vi "MainForMerlin.vi"() -> ()   [LabVIEW 2018]
uses:
  classes/Tushars Events Toolkit/Software/Modules/EventClient_ObjectReference.ctl
  classes/Variable Manager/VariableManager_Bool.vi
  classes/Variable Manager/VariableManager_Double.vi
  <vilib>/Utility/file.llb/Write To Spreadsheet File (string).vi
  classes/Variable Manager/VariableManager_String.vi
  Strict Type Controls/Command.ctl
panel:
  out "filterSetup?":bool
  out "Quit":bool
  out "error out":errorcluster
  in  "error in (no error)":errorcluster
  in  "abort":bool
  in  "start":bool
  out "gratSetup?":bool
  out "statusFilter":bool
  in  "Start Filter":bool
  out "Agilent Current":dbl format="%#.4f A"
  out "Agilent Voltage":dbl format="%#.4f V"
  out "Test Status":bool
  out "statusMerlin":bool
  out "statusMC":bool
  out "statusPS":bool
  out "statusSM":bool
  in  "Start Merlin":bool
  in  "Start Monochromator":bool
  in  "Start Power Supply":bool
  in  "Start Source Meter":bool
  out "Merlin Voltage":dbl format="%#.7f mV"
  out "Measuring Wavelength":dbl format="%#.7f nm"
  out "Source Meter Voltage":dbl format="%#.7f mV"
  in  "Frequency":u32=8 min=8 max=1100 step=1
  in  "setMerlin":bool
  in  "#Filter":enum16{"None", "1 Pole", "2 Pole"}(ring)
  in  "Phase":enum16{"1 Phase", "2 Phase"}(ring)
  in  "SyncMode":T1(ring)
  in  "Time Const":T2(ring)
  in  "tab":T3(tab)=enum."Script"
  in  "exportVT":bool
  out "VTGraph":cluster{dbl[], dbl[]}(graph)
  in  "Test Mode":enum16{"Time Mode", "dV/dt Mode"}(ring)
  in  "Log Interval":u32=50 min=100 step=1 format="%.0f mSec"
  in  "Test Time":dbl step=1.0 format="%<%H:%M:%S>t"
  out "Time Remaining":dbl format="%<%H:%M:%S>t"
  in  "Target dV/dt":dbl format="%#.9f mV"
  in  "Lock In time":dbl step=1.0 format="%<%H:%M:%S>t"
  out "dV/dt":dbl format="%#.11f mV"
  out "Locked Time":dbl step=1.0 format="%<%H:%M:%S>t"
  in  "Perform Test After":T3(ring)=enum."Voltage Vs Wavelength"
  in  "setOffsets":bool
  in  "portD":bool
  in  "portA":bool
  in  "Settling Time (ms)":dbl=5000.0
  in  "To":dbl=1000.0
  in  "Step":dbl=100.0
  in  "From":dbl=100.0
  in  "exportSweep":bool
  out "sweep":cluster{dbl[], dbl[]}[](graph)
  in  "SetSlit":bool
  in  "SetGrating":bool
  in  "setWavelength":bool
  in  "Wavelength":dbl
  in  "Slit":string(combo)
  in  "GratingNo":u8=1 min=1 max=3 step=1
  in  "Sweep Results":i32(listbox)
  in  "exportScriptWave":bool
  out "scriptSweep":cluster{dbl[], dbl[]}[](graph)
  in  "Command":T4
  in  "Parm 4":dbl format="%#.6f"
  in  "Parm 3":dbl format="%#.6f"
  in  "openScript":bool
  in  "exportScript":bool
  in  "update":bool
  out "scriptGraph":cluster{dbl[], dbl[]}(graph)
  in  "Parm 2":dbl format="%#.6f"
  in  "Parm 1":dbl format="%#.6f"
  in  "script":i32(listbox)
  in  "add":bool
  in  "remove":bool
  in  "exportScriptResults":bool
  in  "Script Avg Interval":u32=200 min=100 step=1 format="%.0f mSec"
  # "Status"
  # "Merlin"
  # "Test Type"
  # "Test Time"
  # "Voltage Results"
  # "Monochromator"
  # "Merlin"
  # "Sweep"
  # "NOTE:\n1. if this LED is OFF then GPIB is not connected...\n2. Close program before power off Instruments..."
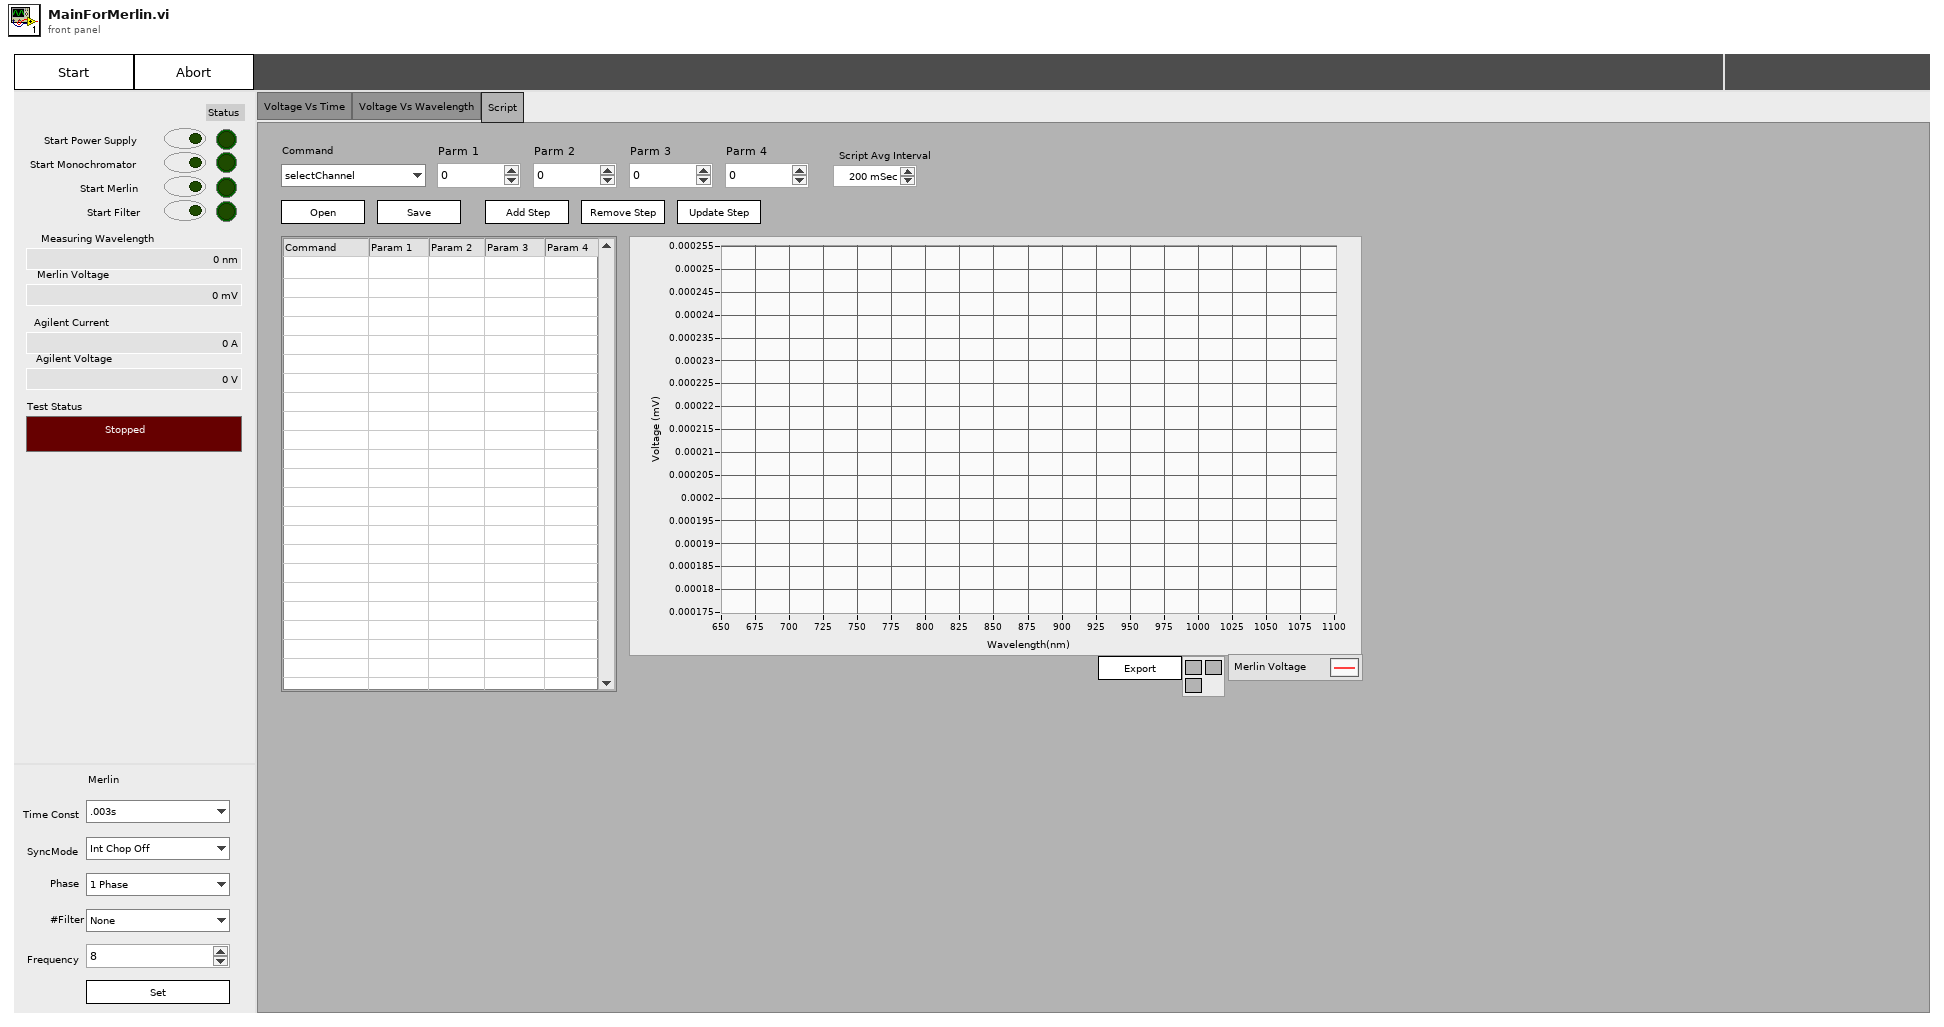
[diagram p1: front panel]
types:
  T1 = enum16{"Int Chop Off", "Int Chop On", "Ext Chop Off", "Ext Chop On"}
  T2 = enum16{".003s", ".010s", ".030s", ".100s", ".300s", "1.00s", "3.00s", "10.0s", "30.0s", "100s"}
  T3 = enum32{"Voltage Vs Time", "Voltage Vs Wavelength", "Script"}
  T4 = typedef "Command.ctl" = enum16{"selectChannel", "setDCVoltage", "setDCCurrent", "setVoltageSteps", "wait", "setWavelength", "setWavelengthSteps"}
  T5 = enum32{"invalid app kind", "Development System", "Run Time System", "Student Edition", "Embedded LabVIEW", "Evaluation", "Custom"}
  T6 = cluster{"startTime":u32, "lastUpdate":u32, "lastVoltage":dbl, "run?":bool, "From":dbl, "time":dbl[], "MerlinVal":dbl[], "SMVolt":dbl[], "sweepType":enum16{"ASC", "DESC"}, "Wavlnth":dbl[], "Test Mode":enum16{"Time Mode", "dV/dt Mode"}, "tab":enum32{"Voltage Vs Time", "Voltage Vs Wavelength", "Script"}, "script":string[][], "dV/dt":dbl[], "graphUpdate":u32}
  T7 = typedef "EventClient_ObjectReference.ctl" = refnum<k1>
  T8 = cluster{"#Stages":enum16{"None", "1 Pole", "2 Pole"}, "Phase":enum16{"1 Phase", "2 Phase"}, "SyncMode":enum16{"Int Chop Off", "Int Chop On", "Ext Chop Off", "Ext Chop On"}, "Time Const":enum16{".003s", ".010s", ".030s", ".100s", ".300s", "1.00s", "3.00s", "10.0s", "30.0s", "100s"}, "Frequency":u32}
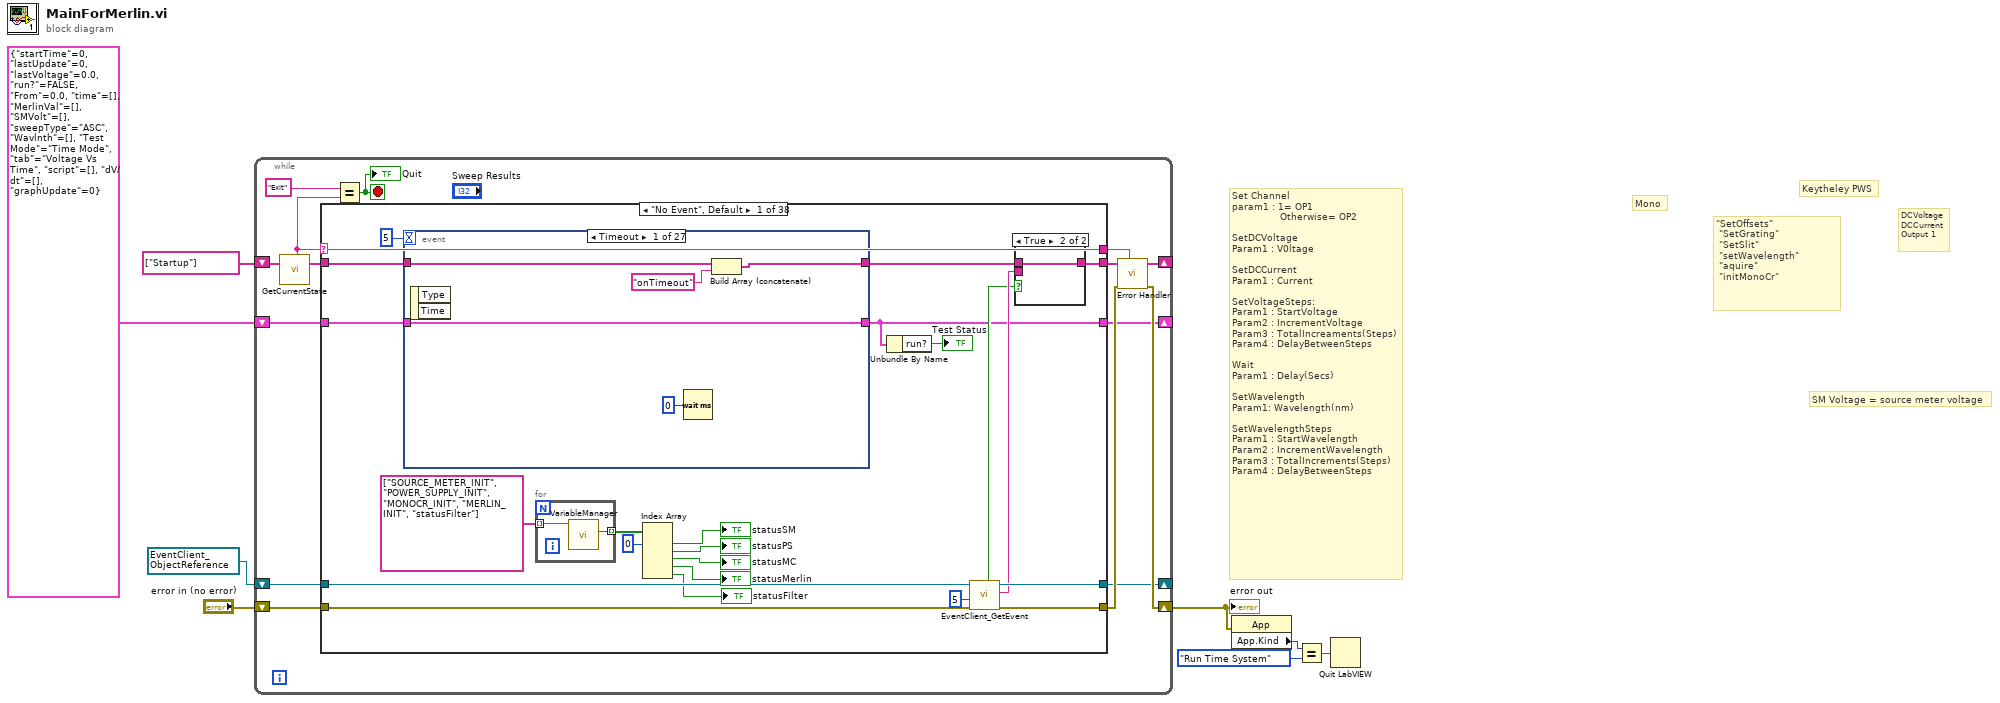
[diagram p0: block diagram]
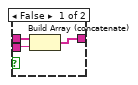
[diagram p2: hidden frame]
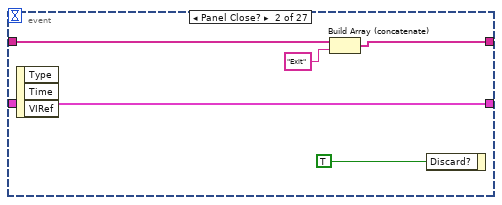
[diagram p3: hidden frame]
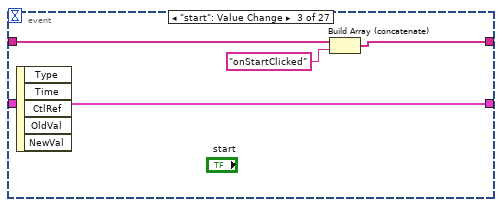
[diagram p4: hidden frame]
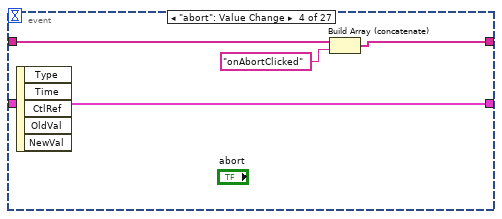
[diagram p5: hidden frame]
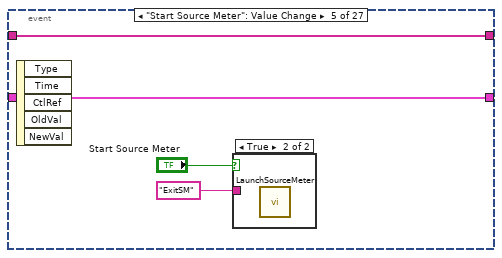
[diagram p6: hidden frame]
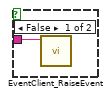
[diagram p7: hidden frame]
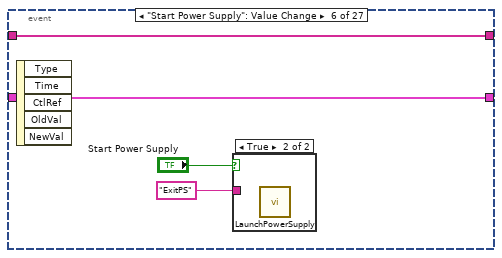
[diagram p8: hidden frame]
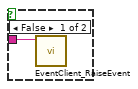
[diagram p9: hidden frame]
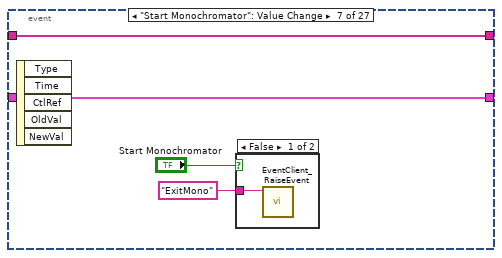
[diagram p10: hidden frame]
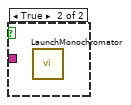
[diagram p11: hidden frame]
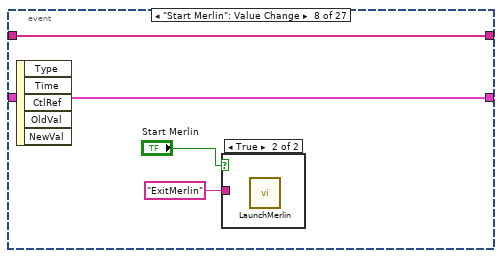
[diagram p12: hidden frame]
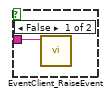
[diagram p13: hidden frame]
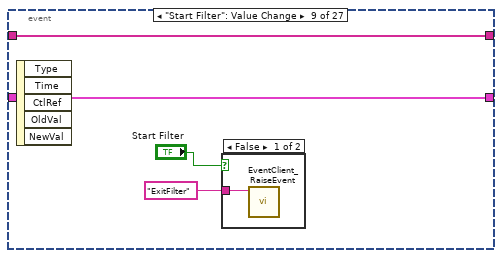
[diagram p14: hidden frame]
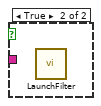
[diagram p15: hidden frame]
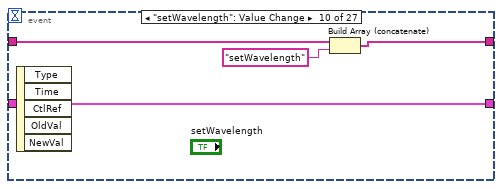
[diagram p16: hidden frame]
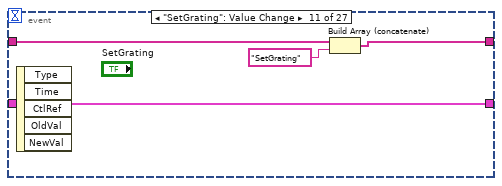
[diagram p17: hidden frame]
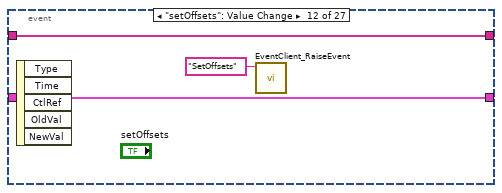
[diagram p18: hidden frame]
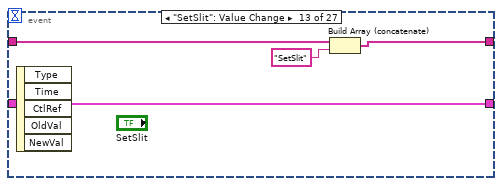
[diagram p19: hidden frame]
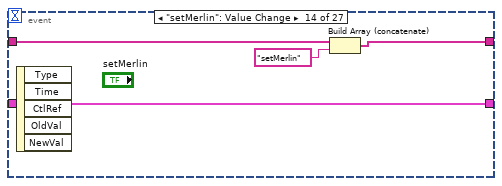
[diagram p20: hidden frame]
diagram:
  w7 = T7 refnum items=["EventClient"] ("reference")
  # "SM Voltage = source meter voltage"
  # "Keytheley PWS"
  # "Mono"
  # "DCVoltage\nDCCurrent\nOutput 1"
  # "\"SetOffsets\"\n \"SetGrating\"  \n \"SetSlit\"\n \"setWavelength\"\n \"aquire\"  \n \"initMonoCr\""
  # "Set Channel\nparam1 : 1= OP1\n                Otherwise= OP2\n\nSetDCVoltage\nParam1 : V0ltage\n\nSetDCCurrent\nParam1 : Current\n\nSetVoltageSteps:\nParam1 : StartVoltage\nParam2 : IncrementVoltage\nParam3 : TotalIncreaments(Steps)\nParam4 : DelayBetweenSteps\n\nWait\nParam1 : Delay(Secs)\n\nSetWavelength\nParam1: Wavelength(nm)\n\nSetWavelengthSteps\nParam1 : StartWavelength\nParam2 : IncrementWavelength\nParam3 : TotalIncrements(Steps)\nParam4 : DelayBetweenSteps"
  n1 = while {
    shift-right: [w19] -> _
    shift-left: string[] ["Startup"] ("State Array Out") -> [w23]
    shift-right: [w15] -> w4
    shift-left: "error in (no error)" -> [w16]
    shift-right: [w12] -> _
    shift-left: w7 -> [w11]
    shift-right: [w9] -> _
    shift-left: T6 {"startTime"=0, "lastUpdate"=0, "lastVoltage"=0.0, "run?"=FALSE, "From"=0.0, "time"=[], "MerlinVal"=[], "SMVolt"=[], "sweepType"=enum."ASC", "Wavlnth"=[], "Test Mode"=enum."Time Mode", "tab"=enum."Voltage Vs Time", "script"=[], "dV/dt"=[], "graphUpdate"=0} -> [w10]
    stop <- w20 stop-if-true
    n2 = call "GetCurrentState.vi"("State Array In"=w23) -> ("Current State"=w13:string, "State Array Out"=w22:string[])  [unwired: 17 in]
    n3 = case shown="\"No Event\", Default" w13 {
      selector: w13 -> [w46 w193 w202 w212 w230 w246 w269 w296 w315 w325 w346 w363 w371 w398 w414 w425 w437 w445 w449 w458 w467 w479 w487 w497 w526 w537 w542 w560 w612 w632 w662 w694 w719 w782 w837 w872 w901 w907]
      tunnel: w22 -> [w45 w192 w208 w213 w231 w247 w270 w297 w302 w326 w347 w364 w372 w399 w415 w426 w438 w446 w453 w462 w469 w483 w488 w498 w527 w538 w543 w551 w595 w616 w654 w686 w710 w783 w838 w873 w900 w904]
      tunnel: [w36 w191 w208 w213 w231 w247 w270 w297 w302 w326 w347 w364 w372 w399 w415 w426 w438 w446 w453 w462 w469 w483 w488 w498 w527 w538 w543 w552 w594 w615 w653 w688 w709 w783 w826 w873 w900 w904] -> w18
      tunnel: [w41 w185 w203 w211 w229 w245 w268 w295 w314 w324 w345 w362 w370 w397 w413 w424 w431 w439 w450 w459 w465 w480 w486 w493 w522 w533 w541 w559 w611 w631 w661 w693 w717 w764 w833 w871 w899 w906] -> w14
      tunnel: [w46 w193 w202 w212 w230 w246 w269 w296 w315 w325 w346 w363 w371 w398 w414 w425 w437 w445 w449 w458 w467 w479 w487 w497 w526 w537 w542 w560 w612 w632 w662 w694 w719 w782 w837 w872 w901 w907] -> w17
      tunnel: w16 -> [w42 w172 w206 w211 w229 w245 w268 w295 w314 w324 w345 w362 w370 w397 w413 w424 w432 w440 w451 w460 w464 w481 w486 w495 w524 w535 w541 w559 w611 w631 w661 w693 w717 w763 w834 w871 w899 w905]
      tunnel: [w40 w183 w205 w210 w228 w244 w267 w294 w313 w323 w344 w361 w369 w396 w412 w423 w436 w444 w452 w461 w468 w482 w485 w491 w520 w531 w540 w558 w610 w630 w660 w692 w718 w781 w836 w870 w898 w902] -> w12
      tunnel: w11 -> [w43 _ w207 w210 w228 w244 w267 w294 w313 w323 w344 w361 w369 w396 w412 w423 w436 w444 w452 w461 w468 w482 w485 w496 w525 w536 w540 w558 w610 w630 w660 w692 w718 w781 w836 w870 w898 w902]
      tunnel: w10 -> [w27 w181 w201 w209 w227 w243 w266 w293 w312 w322 w343 w360 w368 w395 w411 w422 w435 w443 w447 w457 w466 w472 w484 w489 w519 w530 w539 w557 w600 w629 w658 w691 w712 w780 w824 w863 w897 w903]
      tunnel: [w26 w181 w201 w209 w227 w243 w266 w293 w312 w322 w343 w360 w368 w394 w410 w422 w435 w443 w447 w457 w466 w472 w484 w489 w519 w530 w539 w557 w599 w626 w656 w691 w711 w779 w835 w862 w897 w903] -> w9
      frame "No Event", Default {
        n4 = event shown="[0] Timeout" {
          selector: _ -> [_ _ _ _ _ _ _ _ _ _ _ _ _ _ _ _ _ _ _ _ _ _ _ _ _ _ _]
          dyn-events: _ -> [_ _ _ _ _ _ _ _ _ _ _ _ _ _ _ _ _ _ _ _ _ _ _ _ _ _ _]
          timeout: 5 -> [_ _ _ _ _ _ _ _ _ _ _ _ _ _ _ _ _ _ _ _ _ _ _ _ _ _ _]
          tunnel: [w55 w60 w65 w69 w74 w79 w84 w89 w94 w98 w102 w105 w109 w113 w117 w121 w125 w129 w133 w137 w141 w145 w149 w153 w157 w161 w166] -> w37
          tunnel: w45 -> [w57 w62 w66 w70 w74 w79 w84 w89 w94 w99 w103 w105 w110 w114 w118 w122 w126 w130 w134 w138 w142 w146 w150 w154 w158 w162 w166]
          tunnel: w27 -> [w56 w58 w63 w67 w73 w78 w83 w88 w93 w96 w100 w106 w107 w111 w115 w119 w123 w127 w131 w135 w139 w143 w147 w151 w155 w159 w167]
          tunnel: [w56 w58 w63 w67 w73 w78 w83 w88 w93 w96 w100 w106 w107 w111 w115 w119 w123 w127 w131 w135 w139 w143 w147 w151 w155 w159 w167] -> w26
          event Timeout {
            n5 = event-data() -> ()  [unwired: 1 in, 2 out]
            n6 = Wait (ms)(milliseconds to wait=u32 0) -> ()  [unwired: 1 out]
            n7 = Build Array (concatenate)(w57, "onTimeout" ("x")) -> (w55:string[])
          }
          event Panel Close? {
            n8 = event-data() -> ()  [unwired: 1 in, 3 out]
            n9 = Build Array (concatenate)(w62, "Exit" ("x")) -> (w60:string[])
            n10 = event-data("Discard?"=TRUE) -> ()  [unwired: 1 in, 1 out]
          }
          event "start": Value Change {
            n11 = event-data() -> ()  [unwired: 1 in, 5 out]
            n12 = Build Array (concatenate)(w66, "onStartClicked" ("x")) -> (w65:string[])
          }
          event "abort": Value Change {
            n13 = event-data() -> ()  [unwired: 1 in, 5 out]
            n14 = Build Array (concatenate)(w70, "onAbortClicked" ("x")) -> (w69:string[])
          }
          event "Start Source Meter": Value Change {
            n15 = event-data() -> ()  [unwired: 1 in, 5 out]
            n16 = case shown="True" "Start Source Meter" {
              tunnel: "ExitSM" -> [w75 _]
              frame False {
                n17 = call "EventClient_RaiseEvent.vi"("Event"=w75) -> ()  [unwired: 10 in, 1 out]
              }
              frame True {
                n18 = call "LaunchSourceMeter.vi"() -> ()  [unwired: 11 in, 1 out]
              }
            }
          }
          event "Start Power Supply": Value Change {
            n19 = event-data() -> ()  [unwired: 1 in, 5 out]
            n20 = case shown="True" "Start Power Supply" {
              tunnel: "ExitPS" -> [w80 _]
              frame False {
                n21 = call "EventClient_RaiseEvent.vi"("Event"=w80) -> ()  [unwired: 10 in, 1 out]
              }
              frame True {
                n22 = call "LaunchPowerSupply.vi"() -> ()  [unwired: 11 in, 1 out]
              }
            }
          }
          event "Start Monochromator": Value Change {
            n23 = event-data() -> ()  [unwired: 1 in, 5 out]
            n24 = case shown="False" "Start Monochromator" {
              tunnel: "ExitMono" -> [w85 _]
              frame False {
                n25 = call "EventClient_RaiseEvent.vi"("Event"=w85) -> ()  [unwired: 10 in, 1 out]
              }
              frame True {
                n26 = call "LaunchMonochromator.vi"() -> ()  [unwired: 11 in, 1 out]
              }
            }
          }
          event "Start Merlin": Value Change {
            n27 = event-data() -> ()  [unwired: 1 in, 5 out]
            n28 = case shown="True" "Start Merlin" {
              tunnel: "ExitMerlin" -> [w90 _]
              frame False {
                n29 = call "EventClient_RaiseEvent.vi"("Event"=w90) -> ()  [unwired: 10 in, 1 out]
              }
              frame True {
                n30 = call "LaunchMerlin.vi"() -> ()  [unwired: 11 in, 1 out]
              }
            }
          }
          event "Start Filter": Value Change {
            n31 = event-data() -> ()  [unwired: 1 in, 5 out]
            n32 = case shown="False" "Start Filter" {
              tunnel: "ExitFilter" -> [w95 _]
              frame False {
                n33 = call "EventClient_RaiseEvent.vi"("Event"=w95) -> ()  [unwired: 10 in, 1 out]
              }
              frame True {
                n34 = call "LaunchFilter.vi"() -> ()  [unwired: 11 in, 1 out]
              }
            }
          }
          event "setWavelength": Value Change {
            n35 = event-data() -> ()  [unwired: 1 in, 5 out]
            n36 = Build Array (concatenate)(w99, "setWavelength" ("x")) -> (w98:string[])
          }
          event "SetGrating": Value Change {
            n37 = event-data() -> ()  [unwired: 1 in, 5 out]
            n38 = Build Array (concatenate)(w103, "SetGrating" ("x")) -> (w102:string[])
          }
          event "setOffsets": Value Change {
            n39 = event-data() -> ()  [unwired: 1 in, 5 out]
            n40 = call "EventClient_RaiseEvent.vi"("Event"="SetOffsets") -> ()  [unwired: 10 in, 1 out]
          }
          event "SetSlit": Value Change {
            n41 = event-data() -> ()  [unwired: 1 in, 5 out]
            n42 = Build Array (concatenate)(w110, "SetSlit" ("x")) -> (w109:string[])
          }
          event "setMerlin": Value Change {
            n43 = event-data() -> ()  [unwired: 1 in, 5 out]
            n44 = Build Array (concatenate)(w114, "setMerlin" ("x")) -> (w113:string[])
          }
          event "exportSweep": Value Change {
            n45 = event-data() -> ()  [unwired: 1 in, 5 out]
            n46 = Build Array (concatenate)(w118, "exportSweep" ("x")) -> (w117:string[])
          }
          event "exportVT": Value Change {
            n47 = event-data() -> ()  [unwired: 1 in, 5 out]
            n48 = Build Array (concatenate)(w122, "exportVT" ("x")) -> (w121:string[])
          }
          event "portA": Value Change {
            n49 = event-data() -> ()  [unwired: 1 in, 5 out]
            n50 = Build Array (concatenate)(w126, "portA" ("x")) -> (w125:string[])
          }
          event "portD": Value Change {
            n51 = event-data() -> ()  [unwired: 1 in, 5 out]
            n52 = Build Array (concatenate)(w130, "portD" ("x")) -> (w129:string[])
          }
          event "add": Value Change {
            n53 = event-data() -> ()  [unwired: 1 in, 5 out]
            n54 = Build Array (concatenate)(w134, "addStep" ("x")) -> (w133:string[])
          }
          event "remove": Value Change {
            n55 = event-data() -> ()  [unwired: 1 in, 5 out]
            n56 = Build Array (concatenate)(w138, "removeStep" ("x")) -> (w137:string[])
          }
          event "update": Value Change {
            n57 = event-data() -> ()  [unwired: 1 in, 5 out]
            n58 = Build Array (concatenate)(w142, "updateStep" ("x")) -> (w141:string[])
          }
          event "exportScript": Value Change {
            n59 = event-data() -> ()  [unwired: 1 in, 5 out]
            n60 = Build Array (concatenate)(w146, "exportScript" ("x")) -> (w145:string[])
          }
          event "exportScriptResults": Value Change {
            n61 = event-data() -> ()  [unwired: 1 in, 5 out]
            n62 = Build Array (concatenate)(w150, "exportScriptResults" ("x")) -> (w149:string[])
          }
          event "exportScriptWave": Value Change {
            n63 = event-data() -> ()  [unwired: 1 in, 5 out]
            n64 = Build Array (concatenate)(w154, "exportScriptWave" ("x")) -> (w153:string[])
          }
          event "openScript": Value Change {
            n65 = event-data() -> ()  [unwired: 1 in, 5 out]
            n66 = Build Array (concatenate)(w158, "openScript" ("x")) -> (w157:string[])
          }
          event "script": Value Change {
            n67 = event-data() -> ()  [unwired: 1 in, 5 out]
            n68 = Build Array (concatenate)(w162, "onScriptRowSelected" ("x")) -> (w161:string[])
          }
          event Value Change {
            n69 = event-data() -> ("NewVal"=w164:T4)  [unwired: 1 in, 4 out]
            n70 = Index Array(array=string[] ["Set Channel\nparam1 : \n1                 = OP1\nOtherwise = OP2", "SetDCVoltage\nParam1 : V0ltage", "SetDCCurrent\nParam1 : Current", "SetVoltageSteps:\nParam1 : StartVoltage\nParam2 : IncrementVoltage\nParam3 : TotalIncreaments(Steps)\nParam4 : DelayBetweenSteps", "Wait\nParam1 : Delay(Secs)", "SetWavelength\nParam1: Wavelength(nm)", "SetWavelengthSteps\nParam1 : StartWavelength\nParam2 : IncrementWavelength\nParam3 : TotalIncrements(Steps)\nParam4 : DelayBetweenSteps"] ("Array"), index=w164) -> (element=w165:string)
            n71 = property on="Command" class="Enum (strict)"("TipStrip"=w165) -> ()  [unwired: 2 in, 2 out]
          }
        }
        n72 = for {
          tunnel: string[] ["SOURCE_METER_INIT", "POWER_SUPPLY_INIT", "MONOCR_INIT", "MERLIN_INIT", "statusFilter"] ("State Array Out") -> [w48] mode=indexing
          tunnel: [w47] -> w33 mode=indexing
          n73 = call-poly "VariableManager.vi"("Tag"=w48) -> ("Value out"=w47:bool)  [unwired: 7 in, 3 out]
        }
        n74 = Index Array(array=w33, index #1=0 ("index")) -> (element #1=→"statusSM":bool, element #2=→"statusPS":bool, element #3=→"statusMC":bool, element #4=→"statusMerlin":bool, element #5=→"statusFilter":bool)  [unwired: 4 in]
        n75 = Unbundle By Name(w26) -> ("run?"=→"Test Status":bool)
        n76 = call "EventClient_GetEvent.vi"("error in (no error)"=w42, "timeout in ms (-1)"=5, "reference"=w43) -> ("error out"=w41:errorcluster, "Name"=w39:string, "reference out"=w40:T7, "timed out?"=w38:bool)  [unwired: 4 in, 1 out]
        n77 = case shown="True" w38 {
          tunnel: w37 -> [w51 w52]
          tunnel: w39 -> [w50 _]
          tunnel: [w49 w52] -> w36
          frame False {
            n78 = Build Array (concatenate)(w51, w50) -> (w49:string[])
          }
          frame True {
          }
        }
      }
      frame "Startup" {
        w170 = cluster{dbl[], dbl[]}[] [] ("sweep")
        w171 = cluster{dbl[], dbl[]} {[], []} ("VTGraph")
        w175 = string[] ["Command", "Param 1", "Param 2", "Param 3", "Param 4"]  # script
        w176 = FALSE ("Start Source Meter")
        w169 = u32 200 ("Log Interval")
        # "If Multiple instnances of this VI are possible \nthen make sure that client created in each instance gets a different Name"
        n79 = local write "Log Interval"(w169) -> ()
        n80 = local write "Target dV/dt"(1.0 ("Target dV/dt")) -> ()
        n81 = local write "Lock In time"(30.0 ("Lock In time")) -> ()
        n82 = local write "sweep"(w170) -> ()
        n83 = local write "Test Time"(90.0 ("Locked Time")) -> ()
        n84 = local write "VTGraph"(w171) -> ()
        n85 = local write "scriptGraph"(w171) -> ()
        n86 = local write "Script Avg Interval"(w169) -> ()
        n87 = disable-structure shown="Disabled" {
          disable-tunnel: [w200 _] -> w177
          disable-tunnel: w172 -> [w199 _]
          frame Disabled {
            n88 = call "LaunchPowerSupply.vi"("error in (no error)"=w199) -> ("error out"=w198:errorcluster)  [unwired: 10 in]
            n89 = call "LaunchSourceMeter.vi"("error in (no error)"=w198) -> ("error out"=w197:errorcluster)  [unwired: 10 in]
            n90 = call "LaunchMerlin.vi"("error in (no error)"=w197) -> ("error out"=w196:errorcluster)  [unwired: 10 in]
            n91 = call "LaunchMonochromator.vi"("error in (no error)"=w196) -> ("error out"=w200:errorcluster)  [unwired: 10 in]
          }
          frame Enabled {
          }
        }
        n92 = local write "scriptSweep"(w170) -> ()
        n93 = local write "tab"(T3."Voltage Vs Wavelength" ("tab")) -> ()
        n94 = for {
          tunnel: bool[] [FALSE, TRUE] -> [w194] mode=indexing
          i -> [w195]
          n95 = property on="sweep" class="XYGraph (strict)"("Active Plot"=w195, "Plot.Visible?"=w194) -> ()  [unwired: 2 in, 2 out]
          n96 = property on="scriptSweep" class="XYGraph (strict)"("Active Plot"=w195, "Plot.Visible?"=w194) -> ()  [unwired: 2 in, 2 out]
        }
        n97 = Build Array (concatenate)(w192, string[] [] ("State Array Out")) -> (w191:string[])
        n98 = Call Chain() -> (call chain=w189:string[])
        n99 = Index Array(array=w189, index=0) -> (element=w187:string)
        n100 = call "EventClient_Create.vi"("error in (no error)"=w177, "Instance Name"=w187) -> ("error out"=w186:errorcluster, "reference"=w184:T7)  [unwired: 8 in]
        n101 = local write "Start Source Meter"(w176) -> ()
        n102 = local write "Start Power Supply"(w176) -> ()
        n103 = local write "Start Monochromator"(w176) -> ()
        n104 = local write "Start Merlin"(w176) -> ()
        n105 = call "EventClient_SubscribeEvents.vi"("error in (no error)"=w186, "Events"=string[] ["currGrating", "updateScriptSweep"], "reference"=w184) -> ("error out"=w185:errorcluster, "reference out"=w183:T7)  [unwired: 7 in]
        n106 = property on="script" class="MCListbox (strict)"("ColHdrString"=w175, "ItemNames"=string[][] [] ("Item Names")) -> ()  [unwired: 2 in, 2 out]
      }
      frame "Exit" {
        w205 = T7 refnum items=["EventClient"] ("reference out")
        n107 = call "EventClient_Destroy.vi"("error in (no error)"=w206, "reference"=w207) -> ("error out"=w204:errorcluster)  [unwired: 9 in]
        n108 = call "EventClient_RaiseEvent.vi"("error in (no error)"=w204, "Event"=w202) -> ("error out"=w203:errorcluster)  [unwired: 9 in]
      }
      frame "---------------Below are UI Events---------------" {
        # "This State will never Execute\nIt is added just for improving code readability please do not remove this case"
      }
      frame "onScriptRowSelected" {
        w219 = 0 ("index")
        n109 = property on="script" class="MCListbox (strict)"() -> ("ItemNames"=w226:string[][], "Value"=w225:i32)  [unwired: 2 in, 2 out]
        n110 = Index Array(array=w226, index (row)=w225) -> (element=w223:string[])  [unwired: 1 in]
        n111 = Delete From Array(array=w223, index=w219) -> (deleted portion=w222:string, array with subset deleted=w224:string[])  [unwired: 1 in]
        n112 = Scan From String(input string=w222, default 1=Command."selectChannel" ("Command")) -> (output 1=w218:T4)  [unwired: 3 in, 3 out]
        n113 = Fract/Exp String To Number(string=w224) -> (number=w220:dbl[])  [unwired: 3 in, 1 out]
        n114 = Index Array(array=w220, index #1=w219) -> (element #1=w217:dbl, element #2=w216:dbl, element #3=w215:dbl, element #4=w214:dbl)  [unwired: 3 in]
        n115 = local write "Parm 1"(w217) -> ()
        n116 = local write "Parm 2"(w216) -> ()
        n117 = local write "Parm 3"(w215) -> ()
        n118 = local write "Parm 4"(w214) -> ()
        n119 = local write "Command"(w218) -> ()
      }
      frame "exportVT" {
        n120 = local read "VTGraph"() -> (w237:cluster{dbl[], dbl[]})
        n121 = Unbundle(w237) -> (w241:dbl[], w238:dbl[])
        n122 = for {
          tunnel: w241 -> [w252] mode=indexing
          tunnel: "%<%H:%M:%S>t" ("format string") -> [w254]
          tunnel: [w253] -> w240 mode=indexing
          n123 = Format Into String(format string=w254, w252) -> (resulting string=w253:string)  [unwired: 2 in, 1 out]
        }
        n124 = Number To Fractional String(number=w238) -> (F-format string=w239:string[])  [unwired: 3 in]
        n125 = Build Array(w240, w239) -> (w236:string[][])
        n126 = Transpose 2D Array(2D array=w236) -> (transposed array=w232:string[][])
        n127 = call "File Dialog2"("pattern (all files)"="*.csv") -> ("selected path"=w235:path, "error out"=w234:errorcluster)  [unwired: 11 in, 2 out]
        n128 = case shown="Error" w234 {
          selector: w234 -> [_ w251]
          tunnel: w235 -> [w249 _]
          tunnel: w232 -> [w248 _]
          frame No Error {
            n129 = call-poly <vilib>:"Write To Spreadsheet File.vi"("delimiter (\\t)"="," ("delimiter (\\t)"), "2D data"=w248, "file path (dialog if empty)"=w249) -> ()  [unwired: 5 in, 1 out]
          }
          frame Error {
            n130 = call <vilib>:"Clear Errors.vi"("error in (no error)"=w251) -> ()  [unwired: 5 in, 2 out]
          }
        }
      }
      frame "exportScriptResults" {
        n131 = local read "scriptGraph"() -> (w261:cluster{dbl[], dbl[]})
        n132 = Unbundle(w261) -> (w264:dbl[], w260:dbl[])
        n133 = for {
          tunnel: w264 -> [w275] mode=indexing
          tunnel: "%<%H:%M:%S>t" ("format string") -> [w277]
          tunnel: [w276] -> w263 mode=indexing
          n134 = Format Into String(format string=w277, w275) -> (resulting string=w276:string)  [unwired: 2 in, 1 out]
        }
        n135 = Number To Fractional String(number=w260) -> (F-format string=w262:string[])  [unwired: 3 in]
        n136 = Build Array(w263, w262) -> (w259:string[][])
        n137 = Transpose 2D Array(2D array=w259) -> (transposed array=w255:string[][])
        n138 = call "File Dialog3"("pattern (all files)"="*.csv") -> ("selected path"=w258:path, "error out"=w257:errorcluster)  [unwired: 11 in, 2 out]
        n139 = case shown="No Error" w257 {
          selector: w257 -> [_ w274]
          tunnel: w258 -> [w272 _]
          tunnel: w255 -> [w271 _]
          frame No Error {
            n140 = call-poly <vilib>:"Write To Spreadsheet File.vi"("delimiter (\\t)"="," ("delimiter (\\t)"), "2D data"=w271, "file path (dialog if empty)"=w272) -> ()  [unwired: 5 in, 1 out]
          }
          frame Error {
            n141 = call <vilib>:"Clear Errors.vi"("error in (no error)"=w274) -> ()  [unwired: 5 in, 2 out]
          }
        }
      }
      frame "exportScriptWave" {
        (unwired) "%<%H:%M:%S>t" ("format string")
        n142 = local read "scriptSweep"() -> (w290:cluster{dbl[], dbl[]}[])
        n143 = Index Array(array=w290, index #1=0 ("index")) -> (element #1=w289:cluster{dbl[], dbl[]}, element #2=w287:cluster{dbl[], dbl[]})  [unwired: 1 in]
        n144 = Unbundle(w287) -> (w286:dbl[])  [unwired: 1 out]
        n145 = Unbundle(w289) -> (w278:dbl[], w280:dbl[])
        n146 = Number To Fractional String(number=w278) -> (F-format string=w279:string[])  [unwired: 3 in]
        n147 = Number To Fractional String(number=w280) -> (F-format string=w292:string[])  [unwired: 3 in]
        n148 = Number To Fractional String(number=w286) -> (F-format string=w285:string[])  [unwired: 3 in]
        n149 = Build Array(w279, w292, w285) -> (w291:string[][])
        n150 = Transpose 2D Array(2D array=w291) -> (transposed array=w281:string[][])
        n151 = call "File Dialog4"("pattern (all files)"="*.csv") -> ("selected path"=w284:path, "error out"=w283:errorcluster)  [unwired: 11 in, 2 out]
        n152 = case shown="No Error" w283 {
          selector: w283 -> [_ w301]
          tunnel: w284 -> [w299 _]
          tunnel: w281 -> [w298 _]
          frame No Error {
            n153 = call-poly <vilib>:"Write To Spreadsheet File.vi"("delimiter (\\t)"="," ("delimiter (\\t)"), "2D data"=w298, "file path (dialog if empty)"=w299) -> ()  [unwired: 5 in, 1 out]
          }
          frame Error {
            n154 = call <vilib>:"Clear Errors.vi"("error in (no error)"=w301) -> ()  [unwired: 5 in, 2 out]
          }
        }
      }
      frame "openScript" {
        w307 = string[][] []  # script
        n155 = Read from Text File() -> (text=w310:string, error out=w303:errorcluster)  [unwired: 4 in, 2 out]
        n156 = Spreadsheet String To Array(delimiter (Tab)=",", format string="%s", spreadsheet string=w310, array type (2D Dbl)=w307) -> (array=w306:string[][])
        n157 = call <vilib>:"Clear Errors.vi"("error in (no error)"=w303) -> ()  [unwired: 5 in, 2 out]
        n158 = Delete From Array(array=w306, index (row)=0) -> (deleted portion=w304:string[], array with subset deleted=w305:string[][])  [unwired: 2 in]
        n159 = property on="script" class="MCListbox (strict)"("ItemNames"=w305, "ColHdrString"=w304) -> ()  [unwired: 2 in, 2 out]
      }
      frame "exportScript" {
        n160 = property on="script" class="MCListbox (strict)"() -> ("ColHdrString"=w321:string[], "ItemNames"=w320:string[][])  [unwired: 2 in, 2 out]
        n161 = Build Array (concatenate)(w321, w320) -> (w316:string[][])
        n162 = call "File Dialog5"("pattern (all files)"="*.csv") -> ("selected path"=w319:path, "error out"=w318:errorcluster)  [unwired: 11 in, 2 out]
        n163 = case shown="No Error" w318 {
          selector: w318 -> [_ w330]
          tunnel: w319 -> [w328 _]
          tunnel: w316 -> [w327 _]
          frame No Error {
            n164 = call-poly <vilib>:"Write To Spreadsheet File.vi"("delimiter (\\t)"="," ("delimiter (\\t)"), "2D data"=w327, "file path (dialog if empty)"=w328) -> ()  [unwired: 5 in, 1 out]
          }
          frame Error {
            n165 = call <vilib>:"Clear Errors.vi"("error in (no error)"=w330) -> ()  [unwired: 5 in, 2 out]
          }
        }
      }
      frame "addStep" {
        n166 = property on="script" class="MCListbox (strict)"() -> ("ItemNames"=w340:string[][])  [unwired: 2 in, 2 out]
        n167 = Format Into String("Command") -> (resulting string=w336:string)  [unwired: 3 in, 1 out]
        n168 = Build Array("Parm 1", "Parm 2", "Parm 3", "Parm 4") -> (w337:dbl[])
        n169 = Number To Fractional String(number=w337, width (-)=i16 3 ("precision (6)")) -> (F-format string=w335:string[])  [unwired: 2 in]
        n170 = Build Array (concatenate)(w336, w335) -> (w334:string[])
        n171 = Build Array (concatenate)(w340, w334) -> (w339:string[][])
        n172 = property on="script" class="MCListbox (strict)"("ItemNames"=w339) -> ()  [unwired: 2 in, 2 out]
      }
      frame "updateStep" {
        n173 = local read "Command"() -> (w353:T4)
        n174 = local read "Parm 1"() -> (w352:dbl)
        n175 = local read "Parm 2"() -> (w351:dbl)
        n176 = local read "Parm 3"() -> (w349:dbl)
        n177 = local read "Parm 4"() -> (w348:dbl)
        n178 = Format Into String(w353) -> (resulting string=w355:string)  [unwired: 3 in, 1 out]
        n179 = Build Array(w352, w351, w349, w348) -> (w356:dbl[])
        n180 = property on="script" class="MCListbox (strict)"() -> ("ItemNames"=w359:string[][], "Value"=w357:i32)  [unwired: 2 in, 2 out]
        n181 = Number To Fractional String(number=w356) -> (F-format string=w354:string[])  [unwired: 3 in]
        n182 = Build Array (concatenate)(w355, w354) -> (w350:string[])
        n183 = Replace Array Subset(array=w359, new element=w350, index (row)=w357) -> (w358:string[][])  [unwired: 1 in]
        n184 = property on="script" class="MCListbox (strict)"("ItemNames"=w358) -> ()  [unwired: 2 in, 2 out]
      }
      frame "removeStep" {
        n185 = property on="script" class="MCListbox (strict)"() -> ("ItemNames"=w367:string[][], "Value"=w365:i32)  [unwired: 2 in, 2 out]
        n186 = Delete From Array(array=w367, index (row)=w365) -> (array with subset deleted=w366:string[][])  [unwired: 2 in, 1 out]
        n187 = property on="script" class="MCListbox (strict)"("ItemNames"=w366) -> ()  [unwired: 2 in, 2 out]
      }
      frame "onStartClicked" {
        w383 = dbl[] [] ("time")
        n188 = local write "Locked Time"(0.0 ("Locked Time")) -> ()
        n189 = local read "tab"() -> (w378:T3)
        n190 = case shown="\"Script\"" w378 {
          tunnel: [u32 0 u32 0 u32 2000] -> w376
          frame "Voltage Vs Time", Default {
            n191 = local write "VTGraph"(cluster{dbl[], dbl[]} {[], []} ("VTGraph")) -> ()
          }
          frame "Script" {
            n192 = local write "scriptSweep"(cluster{dbl[], dbl[]}[] [] ("scriptSweep")) -> ()
            n193 = local write "scriptGraph"(cluster{dbl[], dbl[]} {[], []} ("scriptGraph")) -> ()
          }
          frame "Voltage Vs Wavelength" {
            n194 = local read "From"() -> (w406:dbl)
            n195 = property on="Sweep Results" class="MCListbox (strict)"("ItemNames"=string[][] [] ("Item Names")) -> ()  [unwired: 2 in, 2 out]
            n196 = local write "sweep"(cluster{dbl[], dbl[]}[] [] ("sweep")) -> ()
            n197 = call "setWavelenght.vi"("wavelength"=w406) -> ()  [unwired: 10 in, 1 out]
          }
        }
        n198 = Wait (ms)(milliseconds to wait=w376) -> ()  [unwired: 1 out]
        n199 = property on="script" class="MCListbox (strict)"() -> ("ItemNames"=w379:string[][])  [unwired: 2 in, 2 out]
        n200 = call-poly "VariableManager.vi"("Operation"=enum16{"Get Tag", "Set Tag"}."Set Tag", "Value"=0.0, "Tag"="measurinWave") -> ()  [unwired: 4 in, 5 out]
        n201 = Less Or Equal?(x="From", y="To") -> (x <= y?=w389:bool)
        n202 = Select(t=enum16{"ASC", "DESC"}."ASC" ("sweepType"), s=w389, f=enum16{"ASC", "DESC"}."DESC" ("sweepType")) -> (s? t:f=w387:enum16{"ASC", "DESC"})
        n203 = Tick Count (ms)() -> (millisecond timer value=w377:u32)
        n204 = call-poly "VariableManager.vi"("Tag"="SM_VOLTAGE" ("String")) -> ("Value out"=w391:dbl)  [unwired: 6 in, 4 out]
        n205 = Bundle By Name(cluster=w395, "graphUpdate"=w377, "startTime"=w377, "lastUpdate"=w377, "run?"=TRUE, "lastVoltage"=w391, "time"=w383, "SMVolt"=w383, "MerlinVal"=w383, "Wavlnth"=w383, "sweepType"=w387, "From"="From", "tab"="tab", "Test Mode"="Test Mode", "script"=w379) -> (w394:T6)
        "Time Remaining" <- "Test Time"
      }
      frame "onAbortClicked" {
        n206 = Bundle By Name(cluster=w411, "run?"=FALSE) -> (w410:T6)
      }
      frame "exportSweep" {
        n207 = property on="Sweep Results" class="MCListbox (strict)"() -> ("ColHdrString"=w420:string[], "ItemNames"=w421:string[][])  [unwired: 2 in, 2 out]
        n208 = Build Array (concatenate)(w420, w421) -> (w416:string[][])
        n209 = call "File Dialog"("pattern (all files)"="*.csv") -> ("selected path"=w419:path, "error out"=w418:errorcluster)  [unwired: 11 in, 2 out]
        n210 = case shown="No Error" w418 {
          selector: w418 -> [_ w430]
          tunnel: w419 -> [w428 _]
          tunnel: w416 -> [w427 _]
          frame No Error {
            n211 = call-poly <vilib>:"Write To Spreadsheet File.vi"("delimiter (\\t)"="," ("delimiter (\\t)"), "2D data"=w427, "file path (dialog if empty)"=w428) -> ()  [unwired: 5 in, 1 out]
          }
          frame Error {
            n212 = call <vilib>:"Clear Errors.vi"("error in (no error)"=w430) -> ()  [unwired: 5 in, 2 out]
          }
        }
      }
      frame "portA" {
        n213 = call "EventClient_RaiseEvent.vi"("error in (no error)"=w432, "Data"="!PORTIN A" ("concatenated string"), "Event"="MerlinWrite") -> ("error out"=w431:errorcluster)  [unwired: 8 in]
      }
      frame "portD" {
        n214 = call "EventClient_RaiseEvent.vi"("error in (no error)"=w440, "Data"="!PORTIN D" ("concatenated string"), "Event"="MerlinWrite") -> ("error out"=w439:errorcluster)  [unwired: 8 in]
      }
      frame "SetGrating" {
        n215 = call "EventClient_RaiseEvent.vi"("error in (no error)"=w451, "Data"="GratingNo", "Event"=w449) -> ("error out"=w450:errorcluster)  [unwired: 8 in]
      }
      frame "SetSlit" {
        n216 = call-poly "VariableManager.vi"("Operation"=enum16{"Get Tag", "Set Tag"}."Set Tag", "Value"="Slit", "Tag"="currSlit") -> ()  [unwired: 5 in, 4 out]
        n217 = call "EventClient_RaiseEvent.vi"("error in (no error)"=w460, "Data"="Slit", "Event"=w458) -> ("error out"=w459:errorcluster)  [unwired: 8 in]
      }
      frame "setWavelength" {
        n218 = call "setWavelenght.vi"("error in (no error)"=w464, "wavelength"="Wavelength") -> ("error out"=w465:errorcluster)  [unwired: 9 in]
      }
      frame "setMerlin" {
        n219 = Bundle By Name(cluster=T8 {"#Stages"=enum."None", "Phase"=enum."1 Phase", "SyncMode"=enum."Int Chop Off", "Time Const"=enum.".003s", "Frequency"=0}, "#Stages"="#Filter", "Phase"="Phase", "SyncMode"="SyncMode", "Time Const"="Time Const", "Frequency"="Frequency") -> (w478:T8)
        n220 = call "EventClient_RaiseEvent.vi"("error in (no error)"=w481, "Data"=w478, "Event"="setMerlin") -> ("error out"=w480:errorcluster)  [unwired: 8 in]
      }
      frame "---------------Below are Menu Events---------------" {
        # "This State will never Execute\nIt is added just for improving code readability please do not remove this case"
      }
      frame "---------------Below are Client Events---------------" {
        # "To Handle Event Duplicate this case. If Event Does not have any data then remove\nGet Event Data and variant to data VIs"
        # "Connect Proper DataType Here"
        n221 = call "EventClient_GetEventData.vi"("error in (no error)"=w495, "reference"=w496) -> ("error out"=w494:errorcluster, "Data"=w492:variant, "reference out"=w491:T7)  [unwired: 7 in]
        n222 = Variant To Data(error in=w494, type=variant, Variant=w492) -> (error out=w493:errorcluster)  [unwired: 1 out]
      }
      frame "updateScriptSweep" {
        n223 = call "EventClient_GetEventData.vi"("error in (no error)"=w524, "reference"=w525) -> ("error out"=w523:errorcluster, "Data"=w521:variant, "reference out"=w520:T7)  [unwired: 7 in]
        n224 = Variant To Data(error in=w523, type=cluster{"wave":dbl, "smV":dbl, "mV":dbl} {"wave"=0.0, "smV"=0.0, "mV"=0.0}, Variant=w521) -> (data=w502:cluster{"wave":dbl, "smV":dbl, "mV":dbl}, error out=w522:errorcluster)
        n225 = local read "scriptSweep"() -> (w504:cluster{dbl[], dbl[]}[])
        n226 = Unbundle By Name(w502) -> ("wave"=w501:dbl, "smV"=w500:dbl, "mV"=w499:dbl)
        n227 = Index Array(array=w504, index #1=0 ("index")) -> (element #1=w506:cluster{dbl[], dbl[]}, element #2=w509:cluster{dbl[], dbl[]})  [unwired: 1 in]
        n228 = Unbundle(w506) -> (w511:dbl[], w512:dbl[])
        n229 = Unbundle(w509) -> (w510:dbl[], w513:dbl[])
        n230 = Build Array (concatenate)(w511, w501) -> (w508:dbl[])
        n231 = Build Array (concatenate)(w512, w500) -> (w516:dbl[])
        n232 = Build Array (concatenate)(w510, w501) -> (w514:dbl[])
        n233 = Build Array (concatenate)(w513, w499) -> (w515:dbl[])
        n234 = Bundle(cluster=w506, w508, w516) -> (w507:cluster{dbl[], dbl[]})
        n235 = Bundle(w514, w515) -> (w517:cluster{dbl[], dbl[]})  [unwired: 1 in]
        n236 = Build Array(w507, w517) -> (→"scriptSweep":cluster{dbl[], dbl[]}[])
      }
      frame "currGrating" {
        n237 = call "EventClient_GetEventData.vi"("error in (no error)"=w535, "reference"=w536) -> ("error out"=w534:errorcluster, "Data"=w532:variant, "reference out"=w531:T7)  [unwired: 7 in]
        n238 = Variant To Data(error in=w534, type=u32 0, Variant=w532) -> (data=w528:u32, error out=w533:errorcluster)
        n239 = local write "GratingNo"(w528) -> ()
      }
      frame "---------------Below are Subroutine states---------------" {
      }
      frame "onTimeout" {
        n240 = Unbundle By Name(w557) -> ("run?"=w556:bool, "tab"=w555:T3, "Test Mode"=w554:enum16{"Time Mode", "dV/dt Mode"}, "lastUpdate"=w553:u32)
        n241 = call-poly "VariableManager.vi"("Tag"="GratingChange?") -> ("Value out"=w548:bool)  [unwired: 7 in, 3 out]
        "gratSetup?" <- w548
        n242 = call-poly "VariableManager.vi"("Tag"="filterChange?") -> ("Value out"=w547:bool)  [unwired: 7 in, 3 out]
        "filterSetup?" <- w547
        n243 = Or(x=w548, y=w547) -> (x .or. y?=w546:bool)
        n244 = case shown="True" w556 {
          tunnel: w555 -> [_ w575]
          tunnel: w554 -> [_ _]
          tunnel: w553 -> [_ w574]
          tunnel: [w568 w571] -> w552
          tunnel: w551 -> [w568 w572]
          tunnel: w546 -> [_ w573]
          frame False {
            n245 = for {
              tunnel: string[] ["SM_VOLTAGE", "MERLIN_VALUE", "DCVoltage", "DCCurrent"] ("State Array Out") -> [w570] mode=indexing
              tunnel: [w569] -> w566 mode=indexing
              n246 = call-poly "VariableManager.vi"("Tag"=w570) -> ("Value out"=w569:dbl)  [unwired: 6 in, 4 out]
            }
            n247 = Index Array(array=w566, index #1=0 ("index")) -> (element #1=→"Source Meter Voltage":dbl, element #2=→"Merlin Voltage":dbl, element #3=→"Agilent Voltage":dbl, element #4=→"Agilent Current":dbl)  [unwired: 3 in]
          }
          frame True {
            n248 = case shown="\"Script\"" w575 {
              tunnel: w574 -> [_ _ _]
              tunnel: w573 -> [_ w579 w586]
              tunnel: w572 -> [w578 w581 w588]
              tunnel: [w576 w580 w587] -> w571
              frame "Voltage Vs Time", Default {
                n249 = Build Array (concatenate)(w578, "accumVTValues" ("String")) -> (w576:string[])
              }
              frame "Voltage Vs Wavelength" {
                n250 = case shown="False" w579 {
                  tunnel: w581 -> [w584 w585]
                  tunnel: [w583 w585] -> w580
                  frame False {
                    n251 = Build Array (concatenate)(w584, "updateSweepGraph" ("String")) -> (w583:string[])
                  }
                  frame True {
                  }
                }
              }
              frame "Script" {
                n252 = case shown="False" w586 {
                  tunnel: w588 -> [w590 w592]
                  tunnel: [w589 w592] -> w587
                  frame False {
                    n253 = Build Array (concatenate)(w590, "executeScript" ("String")) -> (w589:string[])
                  }
                  frame True {
                  }
                }
              }
            }
          }
        }
        n254 = call-poly "VariableManager.vi"("Tag"="measurinWave") -> ("Value out"=→"Measuring Wavelength":dbl)  [unwired: 6 in, 4 out]
      }
      frame "accumVTValues" {
        n255 = Unbundle By Name(w600) -> ("startTime"=w606:u32, "SMVolt"=w602:dbl[], "Test Mode"=w597:enum16{"Time Mode", "dV/dt Mode"})
        n256 = local read "Test Time"() -> (w605:dbl)
        n257 = Tick Count (ms)() -> (millisecond timer value=w607:u32)
        n258 = Subtract(x=w607, y=w606) -> (x-y=w608:u32)
        n259 = call-poly "VariableManager.vi"("Tag"="SM_VOLTAGE") -> ("Value out"=w593:dbl)  [unwired: 6 in, 4 out]
        n260 = Divide(x=w608, y=u32 1000) -> (x/y=w601:dbl)
        n261 = Subtract(x=w605, y=w601) -> (x-y=w604:dbl)
        n262 = Build Array (concatenate)(w602, w593) -> (w598:dbl[])
        n263 = Bundle By Name(cluster=w600, "SMVolt"=w598) -> (w599:T6)
        n264 = case shown="\"Time Mode\", Default" w597 {
          tunnel: w604 -> [w613 _]
          frame "Time Mode", Default {
            n265 = local write "Time Remaining"(w613) -> ()
          }
          frame "dV/dt Mode" {
            n266 = local write "Time Remaining"(0.0 ("Time Remaining")) -> ()
          }
        }
        n267 = Build Array (concatenate)(w595, "updateVTGraph" ("String")) -> (w594:string[])
      }
      frame "updateVTGraph" {
        n268 = Unbundle By Name(w629) -> ("graphUpdate"=w620:u32, "startTime"=w619:u32, "SMVolt"=w628:dbl[], "lastVoltage"=w627:dbl)
        n269 = Tick Count (ms)() -> (millisecond timer value=w621:u32)
        n270 = Subtract(x=w621, y=w619) -> (x-y=w622:u32)
        n271 = Subtract(x=w621, y=w620) -> (x-y=w625:u32)
        n272 = Divide(x=w622, y=u32 1000) -> (x/y=w617:dbl)
        n273 = Greater Or Equal?(x=w625, y="Log Interval") -> (x >= y?=w618:bool)
        n274 = case shown="True" w618 {
          tunnel: w629 -> [w634 w647]
          tunnel: w628 -> [_ w646]
          tunnel: w627 -> [_ w645]
          tunnel: [w634 w642] -> w626
          tunnel: w617 -> [_ w639]
          tunnel: w616 -> [w633 w637]
          tunnel: [w633 w636] -> w615
          frame False {
          }
          frame True {
            w641 = dbl[] [] ("time")
            n275 = call "getAvarageVoltageForInterval.vi"("lastVal"=w645, "voltages"=w646) -> ("avarage"=w638:dbl)  [unwired: 9 in]
            n276 = local write "Source Meter Voltage"(w638) -> ()
            n277 = local read "VTGraph"() -> (w643:cluster{dbl[], dbl[]})
            n278 = Unbundle(w643) -> (w651:dbl[], w650:dbl[])
            n279 = Tick Count (ms)() -> (millisecond timer value=w640:u32)
            n280 = Build Array (concatenate)(w637, "checkForVTAbort" ("String")) -> (w636:string[])
            n281 = Build Array (concatenate)(w651, w639) -> (w649:dbl[])
            n282 = Build Array (concatenate)(w650, w638) -> (w648:dbl[])
            n283 = Bundle By Name(cluster=w647, "time"=w641, "SMVolt"=w641, "graphUpdate"=w640, "lastVoltage"=w638) -> (w642:T6)
            n284 = Bundle(w649, w648) -> (→"VTGraph":cluster{dbl[], dbl[]})  [unwired: 1 in]
          }
        }
      }
      frame "checkForVTAbort" {
        n285 = Unbundle By Name(w658) -> ("Test Mode"=w659:enum16{"Time Mode", "dV/dt Mode"})  [unwired: 1 out]
        n286 = case shown="\"Time Mode\", Default" w659 {
          tunnel: w658 -> [w664 w680]
          tunnel: [w664 w680] -> w657
          tunnel: [w663 w673] -> w655
          frame "Time Mode", Default {
            n287 = local read "Time Remaining"() -> (w665:dbl)
            n288 = Greater Or Equal To 0?(x=w665) -> (x >= 0?=w663:bool)
          }
          frame "dV/dt Mode" {
            n289 = local read "VTGraph"() -> (w672:cluster{dbl[], dbl[]})
            n290 = local read "Log Interval"() -> (w666:u32)
            n291 = local read "Locked Time"() -> (w674:dbl)
            n292 = Unbundle(w672) -> (w670:dbl[], w671:dbl[])
            n293 = call "getdVbydt.vi"("times"=w670, "voltages"=w671) -> ("dV/dT"=w669:dbl)  [unwired: 7 in, 2 out]
            "dV/dt" <- w669
            n294 = Divide(x=w666, y=1000.0 ("x")) -> (x/y=w668:dbl)
            n295 = Less Or Equal?(x=w669, y="Target dV/dt") -> (x <= y?=w679:bool)
            n296 = Add(x=w668, y=w674) -> (x+y=w678:dbl)
            n297 = case shown="True" w679 {
              tunnel: [0.0 ("Locked Time") w682] -> w676
              tunnel: w678 -> [_ w682]
              frame False {
              }
              frame True {
              }
            }
            "Locked Time" <- w676
            n298 = Greater Or Equal?(x="Lock In time", y=w676) -> (x >= y?=w673:bool)
          }
        }
        n299 = Build Array (concatenate)(w654, "checkNextTest" ("String")) -> (w653:string[])
        n300 = Bundle By Name(cluster=w657, "run?"=w655) -> (w656:T6)
      }
      frame "checkNextTest" {
        n301 = Unbundle By Name(w691) -> ("run?"=w690:bool, "tab"=w684:T3)
        n302 = Equal?(x=w684, y="Perform Test After") -> (x = y?=w689:bool)
        n303 = Build Array (concatenate)(w686, "onStartClicked" ("String")) -> (w687:string[])
        n304 = case shown="False" w690 {
          tunnel: w689 -> [w697 _]
          tunnel: w686 -> [w701 w702]
          tunnel: [w700 w702] -> w688
          tunnel: w687 -> [w699 _]
          tunnel: w684 -> [w696 _]
          tunnel: "Perform Test After" -> [w698 _]
          frame False {
            n305 = Select(t=w701, s=w697, f=w699) -> (s? t:f=w700:string[])
            n306 = Select(t=w696, s=w697, f=w698) -> (s? t:f=w695:T3)
            n307 = local write "tab"(w695) -> ()
          }
          frame True {
          }
        }
      }
      frame "updateSweepGraph" {
        n308 = Unbundle By Name(w712) -> ("graphUpdate"=w715:u32)
        n309 = Tick Count (ms)() -> (millisecond timer value=w703:u32)
        n310 = Subtract(x=w703, y=w715) -> (x-y=w716:u32)
        n311 = for {
          tunnel: string[] ["SM_VOLTAGE", "MERLIN_VALUE"] ("State Array Out") -> [w721] mode=indexing
          tunnel: [w720] -> w707 mode=indexing
          n312 = call-poly "VariableManager.vi"("Tag"=w721) -> ("Value out"=w720:dbl)  [unwired: 6 in, 4 out]
        }
        n313 = Greater Or Equal?(x=w716, y="Settling Time (ms)") -> (x >= y?=w713:bool)
        n314 = Index Array(array=w707, index #1=0 ("index")) -> (element #1=w705:dbl, element #2=w704:dbl)  [unwired: 1 in]
        n315 = case shown="False" w713 {
          tunnel: w712 -> [w749 w758]
          tunnel: [w733 w757] -> w711
          tunnel: w710 -> [w750 w759]
          tunnel: [w731 w759] -> w709
          tunnel: w705 -> [_ w752]
          tunnel: w704 -> [_ w751]
          tunnel: w703 -> [w723 _]
          frame True {
            w732 = dbl[] [] ("SMVolt")
            n316 = local read "Measuring Wavelength"() -> (w741:dbl)
            n317 = Unbundle By Name(w749) -> ("SMVolt"=w740:dbl[], "MerlinVal"=w739:dbl[])
            n318 = local read "sweep"() -> (w748:cluster{dbl[], dbl[]}[])
            n319 = Index Array(array=w748, index #1=0 ("index")) -> (element #1=w746:cluster{dbl[], dbl[]}, element #2=w745:cluster{dbl[], dbl[]})  [unwired: 1 in]
            n320 = Unbundle(w746) -> (w744:dbl[], w743:dbl[])
            n321 = Unbundle(w745) -> (w742:dbl[])  [unwired: 1 out]
            n322 = call "AvarageSamples.vi"("samples"=w740) -> ("Avg"=w738:dbl)  [unwired: 10 in]
            n323 = call "AvarageSamples.vi"("samples"=w739) -> ("Avg"=w737:dbl)  [unwired: 10 in]
            n324 = Build Array (concatenate)(w744, w741) -> (w725:dbl[])
            n325 = Build Array (concatenate)(w743, w738) -> (w722:dbl[])
            n326 = Build Array (concatenate)(w742, w737) -> (w724:dbl[])
            n327 = Build Array (concatenate)(w750, "updateSweep") -> (w731:string[])
            n328 = Bundle(w725, w722) -> (w736:cluster{dbl[], dbl[]})  [unwired: 1 in]
            n329 = Bundle(w725, w724) -> (w735:cluster{dbl[], dbl[]})  [unwired: 1 in]
            n330 = Build Array(w725, w722, w724) -> (w728:dbl[][])
            n331 = Bundle By Name(cluster=w749, "SMVolt"=w732, "MerlinVal"=w732, "graphUpdate"=w723) -> (w733:T6)
            n332 = Number To Fractional String(number=w728, width (-)=i16 7) -> (F-format string=w727:string[][])  [unwired: 2 in]
            n333 = Build Array(w736, w735) -> (→"sweep":cluster{dbl[], dbl[]}[])
            n334 = Transpose 2D Array(2D array=w727) -> (transposed array=w726:string[][])
            n335 = property on="Sweep Results" class="MCListbox (strict)"("ItemNames"=w726) -> ()  [unwired: 2 in, 2 out]
          }
          frame False {
            n336 = Unbundle By Name(w758) -> ("SMVolt"=w756:dbl[], "MerlinVal"=w755:dbl[])
            n337 = Build Array (concatenate)(w756, w752) -> (w754:dbl[])
            n338 = Build Array (concatenate)(w755, w751) -> (w753:dbl[])
            n339 = Bundle By Name(cluster=w758, "SMVolt"=w754, "MerlinVal"=w753) -> (w757:T6)
          }
        }
        n340 = local write "Merlin Voltage"(w704) -> ()
        n341 = local write "Source Meter Voltage"(w705) -> ()
      }
      frame "updateSweep" {
        n342 = Unbundle By Name(w780) -> ("SMVolt"=w778:dbl[], "MerlinVal"=w777:dbl[], "sweepType"=w769:enum16{"ASC", "DESC"}, "From"=w768:dbl)
        n343 = local read "To"() -> (w766:dbl)
        n344 = case shown="\"ASC\"" w769 {
          tunnel: w768 -> [w806 w811]
          tunnel: "Step" -> [w810 w815]
          tunnel: [w809 w814] -> w761
          tunnel: w766 -> [w808 w813]
          tunnel: [w807 w812] -> w765
          tunnel: [w806 w811] -> w762
          frame "DESC" {
            n345 = Subtract(x=w806, y=w810) -> (x-y=w809:dbl)
            n346 = Less Or Equal?(x=w808, y=w806) -> (x <= y?=w807:bool)
          }
          frame "ASC" {
            n347 = Add(x=w811, y=w815) -> (x+y=w814:dbl)
            n348 = Greater Or Equal?(x=w813, y=w811) -> (x >= y?=w812:bool)
          }
        }
        n349 = local read "From"() -> (w760:dbl)
        n350 = case shown="False" w765 {
          tunnel: w763 -> [w802 w805]
          tunnel: [w801 w804] -> w764
          tunnel: w762 -> [_ w803]
          tunnel: w760 -> [w784 _]
          frame False {
            w790 = 0 ("index (row)")
            n351 = local read "sweep"() -> (w798:cluster{dbl[], dbl[]}[])
            n352 = call "setWavelenght.vi"("error in (no error)"=w802, "wavelength"=w784) -> ("error out"=w801:errorcluster)  [unwired: 9 in]
            n353 = property on="Sweep Results" class="MCListbox (strict)"() -> ("ItemNames"=w800:string[][])  [unwired: 2 in, 2 out]
            n354 = Index Array(array=w798, index #1=0 ("index")) -> (element #1=w796:cluster{dbl[], dbl[]}, element #2=w795:cluster{dbl[], dbl[]})  [unwired: 1 in]
            n355 = Unbundle(w796) -> (w793:dbl[], w791:dbl[])
            n356 = Unbundle(w795) -> (w792:dbl[])  [unwired: 1 out]
            n357 = Delete From Array(array=w800, index (row)=w790) -> (array with subset deleted=w799:string[][])  [unwired: 2 in, 1 out]
            n358 = Delete From Array(array=w793, index=w790) -> (array with subset deleted=w789:dbl[])  [unwired: 1 in, 1 out]
            n359 = Delete From Array(array=w791, index=w790) -> (array with subset deleted=w788:dbl[])  [unwired: 1 in, 1 out]
            n360 = Delete From Array(array=w792, index=w790) -> (array with subset deleted=w787:dbl[])  [unwired: 1 in, 1 out]
            n361 = Bundle(w789, w788) -> (w786:cluster{dbl[], dbl[]})  [unwired: 1 in]
            n362 = Bundle(w789, w787) -> (w785:cluster{dbl[], dbl[]})  [unwired: 1 in]
            n363 = property on="Sweep Results" class="MCListbox (strict)"("ItemNames"=w799) -> ()  [unwired: 2 in, 2 out]
            n364 = Build Array(w786, w785) -> (w794:cluster{dbl[], dbl[]}[])
            n365 = local write "sweep"(w794) -> ()
          }
          frame True {
            n366 = call "setWavelenght.vi"("error in (no error)"=w805, "wavelength"=w803) -> ("error out"=w804:errorcluster)  [unwired: 9 in]
          }
        }
        n367 = for {
          tunnel: string[] ["SM_VOLTAGE", "MERLIN_VALUE"] ("State Array Out") -> [w817] mode=indexing
          tunnel: [w816] -> w773 mode=indexing
          n368 = call-poly "VariableManager.vi"("Tag"=w817) -> ("Value out"=w816:dbl)  [unwired: 6 in, 4 out]
        }
        n369 = Index Array(array=w773, index #1=0 ("index")) -> (element #1=w771:dbl, element #2=w770:dbl)  [unwired: 1 in]
        n370 = Build Array (concatenate)(w778, w771) -> (w776:dbl[])
        n371 = Build Array (concatenate)(w777, w770) -> (w775:dbl[])
        n372 = Bundle By Name(cluster=w780, "SMVolt"=w776, "MerlinVal"=w775, "run?"=w765, "From"=w761) -> (w779:T6)
      }
      frame "executeScript" {
        n373 = for {
          tunnel: string[] ["DCVoltage", "DCCurrent", "SM_VOLTAGE"] ("State Array Out") -> [w854] mode=indexing
          tunnel: [w853] -> w830 mode=indexing
          n374 = call-poly "VariableManager.vi"("Tag"=w854) -> ("Value out"=w853:dbl)  [unwired: 6 in, 4 out]
        }
        n375 = Unbundle By Name(w824) -> ("script"=w820:string[][], "lastUpdate"=w832:u32)
        n376 = Index Array(array=w830, index #1=0 ("index")) -> (element #1=w827:dbl, element #2=w828:dbl, element #3=w822:dbl)  [unwired: 2 in]
        n377 = call "executeScript.vi"("script"=w820, "lastUpdate"=w832, "error in (no error)"=w834) -> ("scriptOut"=w819:string[][], "lastUpdate 2"=w823:u32, "error out"=w833:errorcluster)  [unwired: 5 in]
        n378 = local write "Source Meter Voltage"(w822) -> ()
        n379 = local write "Agilent Current"(w828) -> ()
        n380 = local write "Agilent Voltage"(w827) -> ()
        n381 = Empty Array?(array=w819) -> (empty?=w821:bool)
        n382 = Not(x=w821) -> (.not. x?=w818:bool)
        n383 = Bundle By Name(cluster=w824, "script"=w819, "lastUpdate"=w823, "run?"=w818) -> (w835:T6)
        n384 = case shown="False" w818 {
          frame False {
            w847 = 0 ("index (row)")
            n385 = local read "scriptSweep"() -> (w839:cluster{dbl[], dbl[]}[])
            n386 = Index Array(array=w839, index #1=0 ("index")) -> (element #1=w841:cluster{dbl[], dbl[]}, element #2=w842:cluster{dbl[], dbl[]})  [unwired: 1 in]
            n387 = Unbundle(w841) -> (w844:dbl[], w846:dbl[])
            n388 = Unbundle(w842) -> (w845:dbl[])  [unwired: 1 out]
            n389 = Delete From Array(array=w844, index=w847) -> (array with subset deleted=w848:dbl[])  [unwired: 1 in, 1 out]
            n390 = Delete From Array(array=w846, index=w847) -> (array with subset deleted=w849:dbl[])  [unwired: 1 in, 1 out]
            n391 = Delete From Array(array=w845, index=w847) -> (array with subset deleted=w850:dbl[])  [unwired: 1 in, 1 out]
            n392 = Bundle(w848, w849) -> (w851:cluster{dbl[], dbl[]})  [unwired: 1 in]
            n393 = Bundle(w848, w850) -> (w852:cluster{dbl[], dbl[]})  [unwired: 1 in]
            n394 = Build Array(w851, w852) -> (w843:cluster{dbl[], dbl[]}[])
            n395 = local write "scriptSweep"(w843) -> ()
          }
          frame True {
          }
        }
        n396 = Build Array (concatenate)(w838, "updateScriptGraph" ("String")) -> (w826:string[])
      }
      frame "updateScriptGraph" {
        n397 = Unbundle By Name(w863) -> ("startTime"=w867:u32, "time"=w861:dbl[], "SMVolt"=w860:dbl[], "graphUpdate"=w855:u32)
        n398 = call-poly "VariableManager.vi"("Tag"="SM_VOLTAGE" ("String")) -> ("Value out"=w857:dbl)  [unwired: 6 in, 4 out]
        n399 = Tick Count (ms)() -> (millisecond timer value=w856:u32)
        n400 = Subtract(x=w856, y=w855) -> (x-y=w866:u32)
        n401 = Subtract(x=w856, y=w867) -> (x-y=w869:u32)
        n402 = Greater Or Equal?(x=w866, y="Script Avg Interval") -> (x >= y?=w864:bool)
        n403 = Divide(x=w869, y=u32 1000) -> (x/y=w859:dbl)
        n404 = case shown="True" w864 {
          tunnel: w861 -> [w881 _]
          tunnel: w860 -> [w880 w892]
          tunnel: w859 -> [w879 w888]
          tunnel: w857 -> [w878 w886]
          tunnel: w863 -> [w877 w891]
          tunnel: [w876 w890] -> w862
          tunnel: w856 -> [_ w889]
          frame False {
            n405 = Build Array (concatenate)(w881, w879) -> (w875:dbl[])
            n406 = Build Array (concatenate)(w880, w878) -> (w874:dbl[])
            n407 = Bundle By Name(cluster=w877, "time"=w875, "SMVolt"=w874) -> (w876:T6)
          }
          frame True {
            w884 = dbl[] []
            # "smV/Time\nmerlinV/wavelen\nsmV/wavelen"
            n408 = local read "scriptGraph"() -> (w883:cluster{dbl[], dbl[]})
            n409 = Build Array (concatenate)(w892, w886) -> (w887:dbl[])
            n410 = Unbundle(w883) -> (w896:dbl[], w893:dbl[])
            n411 = call "AvarageSamples.vi"("samples"=w887) -> ("Avg"=w885:dbl)  [unwired: 10 in]
            n412 = Build Array (concatenate)(w896, w888) -> (w895:dbl[])
            n413 = Build Array (concatenate)(w893, w885) -> (w894:dbl[])
            n414 = Bundle By Name(cluster=w891, "graphUpdate"=w889, "time"=w884, "SMVolt"=w884) -> (w890:T6)
            n415 = Bundle(cluster=w883, w895, w894) -> (→"scriptGraph":cluster{dbl[], dbl[]})
          }
        }
      }
      frame "---------------Below are Error Handling VIs---------------" {
      }
      frame "Error" {
        n416 = disable-structure shown="Disabled" {
          disable-tunnel: [errorcluster {"status"=FALSE, "code"=0, "source"=""} ("error in (no error)") _] -> w906
          disable-tunnel: w905 -> [w908 _]
          frame Disabled {
            n417 = Call Chain() -> (call chain=w915:string[])
            n418 = for {
              tunnel: w915 -> [w922] mode=indexing
              shift-right: [w920] -> w912
              shift-left: "" -> [w923]
              n419 = Concatenate Strings(w923, w922, " -> ") -> (w920:string)
            }
            n420 = Unbundle By Name(w908) -> ("code"=w910:i32, "source"=w909:string)
            n421 = Match Pattern(string=w909, regular expression=":") -> (before substring=w913:string, after substring=w917:string)  [unwired: 1 in, 2 out]
            n422 = Format Into String(format string="Error Occured In\"%s\" state of \"%s\" VI\nError Code: %d\nError Description: \"%s\"", w913, w912, w910, w917) -> (resulting string=w916:string)  [unwired: 2 in, 1 out]
            n423 = One Button Dialog(message=w916) -> ()  [unwired: 1 in, 1 out]
          }
          frame Enabled {
          }
        }
      }
    }
    n424 = Equal?(x="Exit", y=w13) -> (x = y?=w20:bool)
    "Quit" <- w20
    n425 = call "Error Handler.vi"("Current State"=w17, "error in (no error)"=w14, "Msg Queue In"=w18) -> ("error out"=w15:errorcluster, "Msg Queue Out"=w19:string[])  [unwired: 7 in]
  }
  "error out" <- w4
  n426 = property class="App"(error in=w4) -> ("App.Kind"=w3:T5)  [unwired: 1 in, 2 out]
  n427 = Equal?(x=w3, y=T5."Run Time System") -> (x = y?=w1:bool)
  n428 = Quit LabVIEW(quit? (T)=w1) -> ()
